vi "XML Script - Control (Variant Typedef).vi"(0 "indicator?":bool, 1 "prefix (name)":string, 2 "in":i32=-1, 3 "label":string, 5 "name":string, 7 "vi path":path, 9 "type index":i32=-1, 11 "x":i32=-1, 12 "y":i32=-1, 13 "out":i32=-1, 14 "conpane index":i32=-1) -> (6 "XML Script Command - Control":string, 8 "name (wire source)":string)   [LabVIEW 2017]
uses:
  <vilib>/_script/XML Scripting/XML Script Attribute.ctl
  <vilib>/_script/XML Scripting/XML Script Tag.ctl
  <vilib>/_script/XML Scripting/XML Script - PathToXMLString.vi
panel:
  # "position"
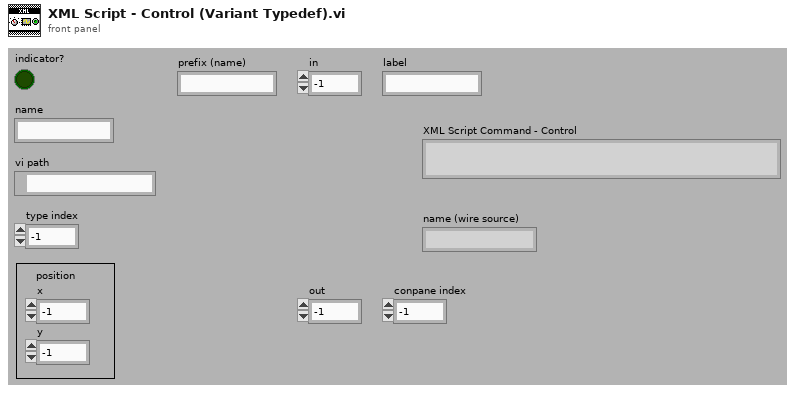
[diagram p1: front panel]
types:
  T1 = typedef "XML Script Attribute.ctl" = enum16{"name", "style", "path", "position", "in", "out", "width", "height", "index", "value", "default", "location", "offset", "typeindex", "size", "source", "destination", "indicator", "type", "controlname", "label", "conpaneidx", "mode", "description", "hasCondTerm", "linkIdentity", "caseselectortype", "concatInputs", "inName", "instantiationpath", "loopCondition", "IndexMode", "formulaInputs", "formulaOutputs", "msnFuncName", "msnIsDynamic", "msnIsODEUserFunction", "ignoreSearchDialog"}
  T2 = typedef "XML Script Tag.ctl" = enum16{"Script", "Function", "SubVI", "GrowableFunction", "Structure", "MultiframeStructure", "Frame", "Tunnel", "ShiftRegister", "Constant", "Control", "Terminal", "Wire", "StaticVIReference", "ControlTerminal", "CompoundArithmetic", "FlatSequence", "FlatSequenceFrame", "MathScriptCallByRef", "BuildArray", "GenericSubVI", "MathScriptNode"}
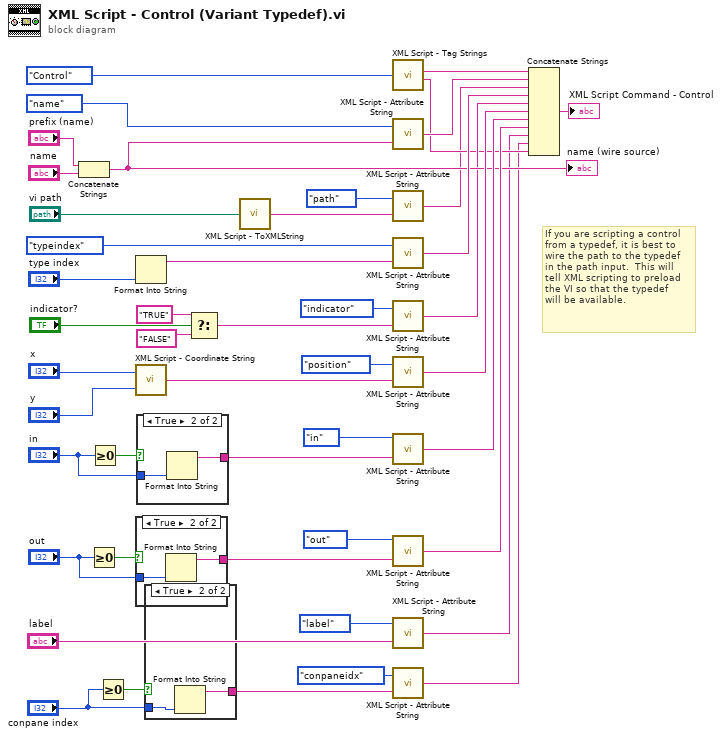
[diagram p0: block diagram]
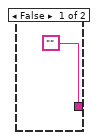
[diagram p2: hidden frame]
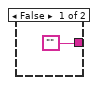
[diagram p3: hidden frame]
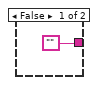
[diagram p4: hidden frame]
diagram:
  # "If you are scripting a control\nfrom a typedef, it is best to\nwire the path to the typedef\nin the path input.  This will\ntell XML scripting to preload\nthe VI so that the typedef\nwill be available."
  n1 = Concatenate Strings("prefix (name)", "name") -> (w22:string)
  "name (wire source)" <- w22
  n2 = Greater Or Equal To 0?(x="out") -> (x >= 0?=w34:bool)
  n3 = Greater Or Equal To 0?(x="in") -> (x >= 0?=w25:bool)
  n4 = Greater Or Equal To 0?(x="conpane index") -> (x >= 0?=w9:bool)
  n5 = Format Into String("type index") -> (resulting string=w28:string)  [unwired: 3 in, 1 out]
  n6 = call <vilib>:"XML Script - Coordinate String.vi"("y"="y", "x"="x") -> ("(x,y)"=w43:string)
  n7 = case shown="True" w34 {
    tunnel: "out" -> [_ w49]
    tunnel: ["" w48] -> w31
    frame False {
    }
    frame True {
      n8 = Format Into String(w49) -> (resulting string=w48:string)  [unwired: 3 in, 1 out]
    }
  }
  n9 = case shown="True" w25 {
    tunnel: "in" -> [_ w52]
    tunnel: ["" w51] -> w27
    frame False {
    }
    frame True {
      n10 = Format Into String(w52) -> (resulting string=w51:string)  [unwired: 3 in, 1 out]
    }
  }
  n11 = case shown="True" w9 {
    tunnel: "conpane index" -> [_ w55]
    tunnel: ["" w54] -> w7
    frame False {
    }
    frame True {
      n12 = Format Into String(w55) -> (resulting string=w54:string)  [unwired: 3 in, 1 out]
    }
  }
  n13 = Select(t="TRUE", s="indicator?", f="FALSE") -> (s? t:f=w16:string)
  n14 = call-poly <vilib>:"XML Script - ToXMLString.vi"("Path"="vi path") -> ("Valid XML String (out)"=w4:string)
  n15 = call <vilib>:"XML Script - Tag Strings.vi"("XML Script Tag"=XML_Script_Tag."Control") -> ("XML String - Begin Tag"=w40:string, "XML String - End Tag"=w11:string)  [unwired: 2 in]
  n16 = call <vilib>:"XML Script - Attribute String.vi"("Attribute String"=w22, "XML Script Attribute"=XML_Script_Attribute."name") -> ("XML Script - Attribute String"=w38:string)
  n17 = call <vilib>:"XML Script - Attribute String.vi"("Attribute String"=w4, "XML Script Attribute"=XML_Script_Attribute."path") -> ("XML Script - Attribute String"=w1:string)
  n18 = call <vilib>:"XML Script - Attribute String.vi"("Attribute String"=w28, "XML Script Attribute"=XML_Script_Attribute."typeindex") -> ("XML Script - Attribute String"=w36:string)
  n19 = call <vilib>:"XML Script - Attribute String.vi"("Attribute String"=w16, "XML Script Attribute"=XML_Script_Attribute."indicator") -> ("XML Script - Attribute String"=w14:string)
  n20 = call <vilib>:"XML Script - Attribute String.vi"("Attribute String"=w43, "XML Script Attribute"=XML_Script_Attribute."position") -> ("XML Script - Attribute String"=w35:string)
  n21 = call <vilib>:"XML Script - Attribute String.vi"("Attribute String"=w27, "XML Script Attribute"=XML_Script_Attribute."in") -> ("XML Script - Attribute String"=w23:string)
  n22 = call <vilib>:"XML Script - Attribute String.vi"("Attribute String"=w31, "XML Script Attribute"=XML_Script_Attribute."out") -> ("XML Script - Attribute String"=w30:string)
  n23 = call <vilib>:"XML Script - Attribute String.vi"("Attribute String"="label", "XML Script Attribute"=XML_Script_Attribute."label") -> ("XML Script - Attribute String"=w10:string)
  n24 = call <vilib>:"XML Script - Attribute String.vi"("Attribute String"=w7, "XML Script Attribute"=XML_Script_Attribute."conpaneidx") -> ("XML Script - Attribute String"=w6:string)
  n25 = Concatenate Strings(w40, w38, w1, w36, w14, w35, w23, w30, w10, w6, w11) -> (→"XML Script Command - Control":string)
